vi "hw3p5_hickey.vi"() -> ()   [LabVIEW 2014]
panel:
  out "Array":dbl[](array[numeric])
  in  "N":i32
  out "Waveform Graph":u32[](graph)
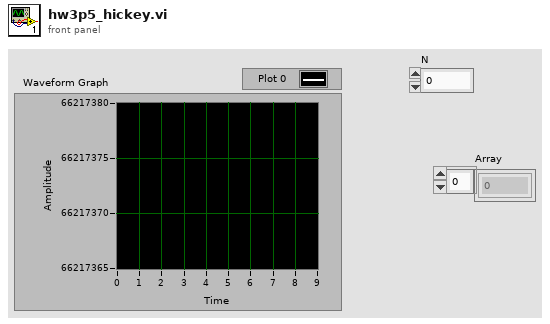
[diagram p1: front panel]
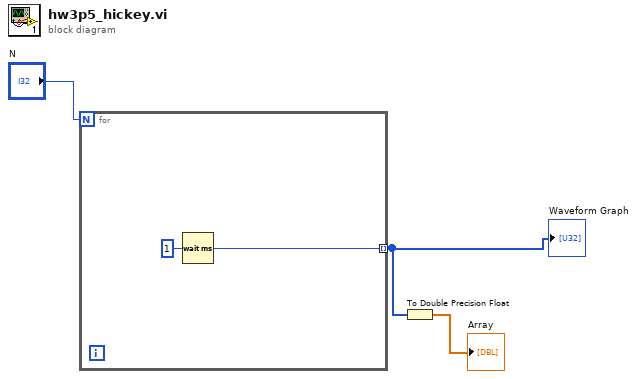
[diagram p0: block diagram]
diagram:
  n1 = for {
    N: "N" -> [_]
    tunnel: [w4] -> w1 mode=indexing
    n2 = Wait (ms)(milliseconds to wait=u32 1) -> (millisecond timer value=w4:u32)
  }
  "Waveform Graph" <- w1
  n3 = To Double Precision Float(number=w1) -> (double precision float=→"Array":dbl[])
